vi "Wait.vi"() -> ()   [LabVIEW 2017]
uses:
  Framework/Robot Global Data.vi
panel:
  in  "Time":dbl
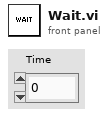
[diagram p1: front panel]
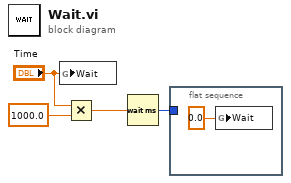
[diagram p0: block diagram]
diagram:
  n1 = global write "Robot Global Data.vi" "Wait"("Time") -> ()
  n2 = Multiply(x="Time", y=1000.0) -> (x*y=w3:dbl)
  n3 = Wait (ms)(milliseconds to wait=w3) -> (millisecond timer value=w2:u32)
  n4 = flat-sequence {
    tunnel: w2 -> [_]
    frame #0 {
      n5 = global write "Robot Global Data.vi" "Wait"(0.0 ("Wait")) -> ()
    }
  }
